vi "三角函數功能.vi"() -> ()   [LabVIEW 2015]
panel:
  out "angle":dbl(graph)
  out "Numeric":i32
  out "Boolean":bool
  out "radian":dbl(graph)
  in  "angle Control 2":dbl
  in  "三角函數":u16(ring)=1 items=["sin", "cos", "tan", "csc", "sec", "cot"]
  out "res angle(num)":dbl
  in  "Stop Button":bool
  out "換算角度 angle (num)":dbl
  in  "angle Control":dbl(slide) scale=0.0..360.0
  out "res radian(num)":dbl
  out "res angle(gauge)":dbl(knob)
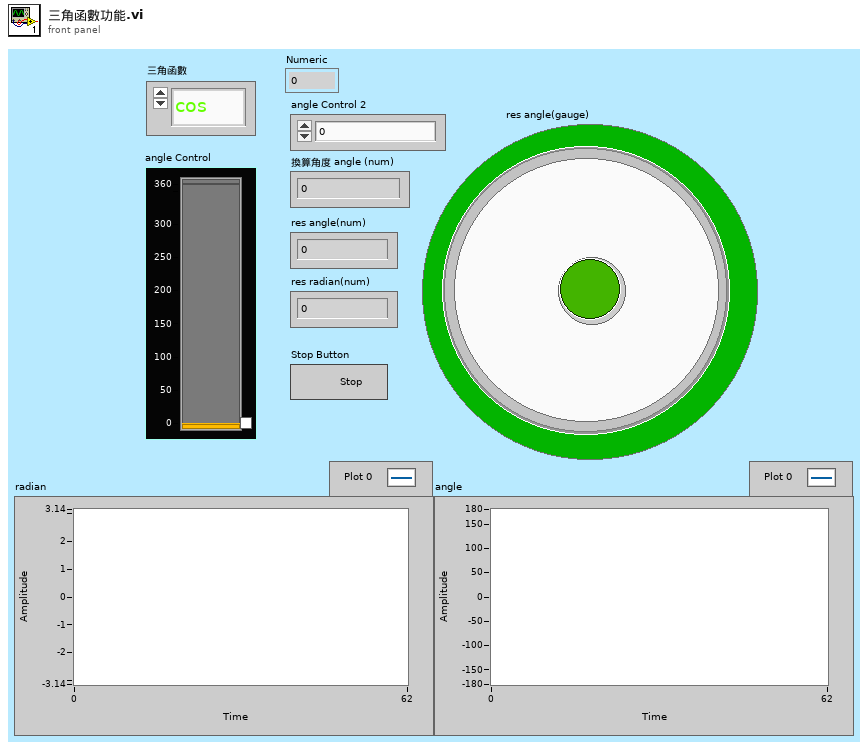
[diagram p1: front panel]
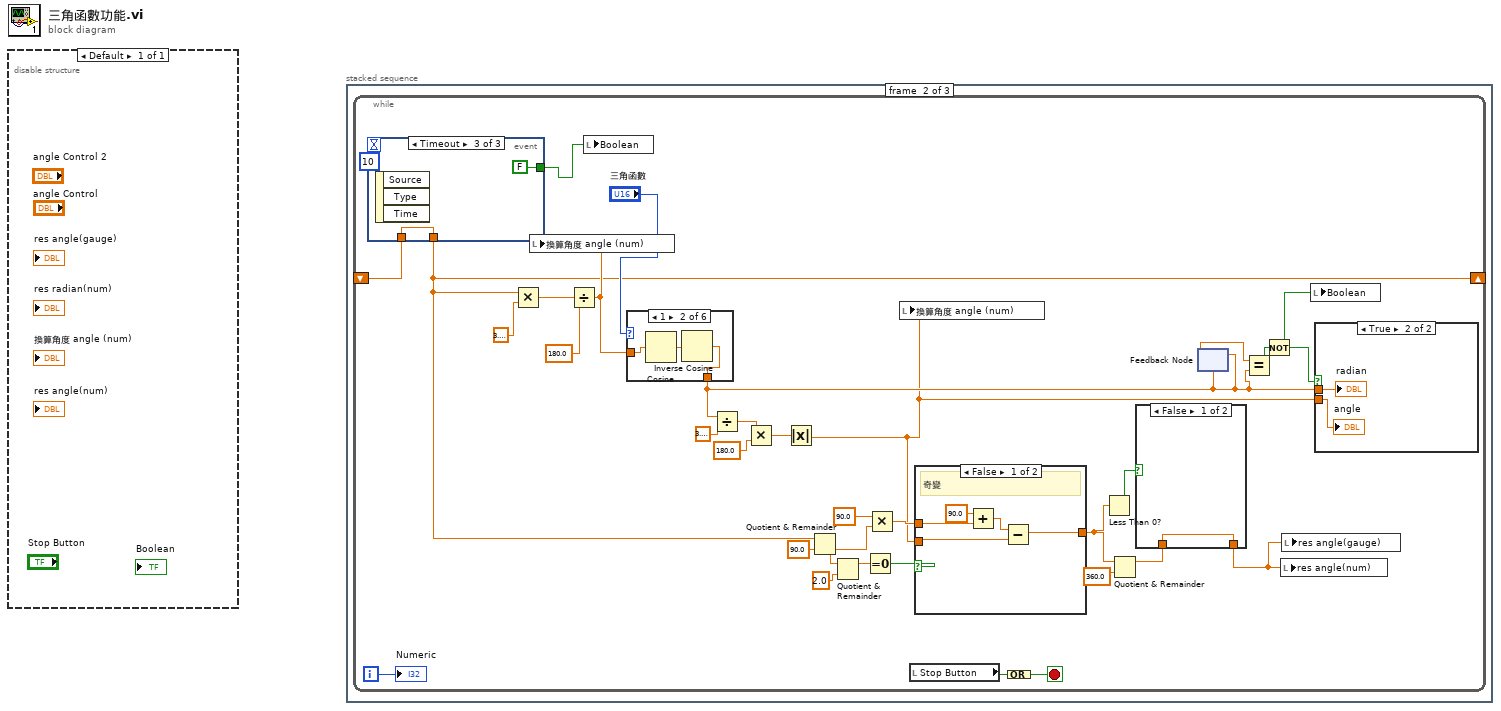
[diagram p0: block diagram]
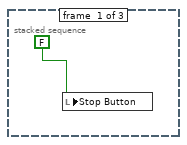
[diagram p2: hidden frame]
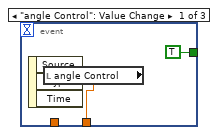
[diagram p3: hidden frame]
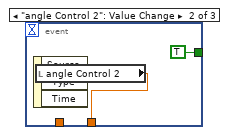
[diagram p4: hidden frame]
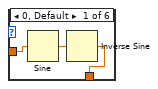
[diagram p6: hidden frame]
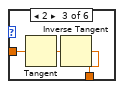
[diagram p7: hidden frame]
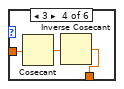
[diagram p8: hidden frame]
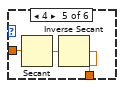
[diagram p9: hidden frame]
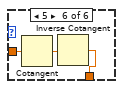
[diagram p10: hidden frame]
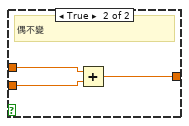
[diagram p12: hidden frame]
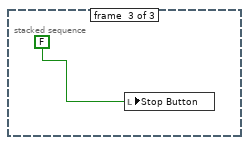
[diagram p13: hidden frame]
diagram:
  n1 = disable-structure shown="Default" {
    frame Enabled {
    }
  }
  n2 = stacked-sequence {
    frame #0 {
      n3 = local write "Stop Button"(FALSE ("Stop Button")) -> ()
    }
    frame #1 {
      n4 = while {
        shift-right: [w4] -> _
        shift-left: _ -> [w3]
        i -> [w6]
        stop <- w34 stop-if-true
        n5 = event shown="[2] Timeout" {
          selector: _ -> [_ _ _]
          dyn-events: _ -> [_ _ _]
          timeout: 10 -> [_ _ _]
          tunnel: [w36 w38 w39] -> w4
          tunnel: [TRUE TRUE FALSE] -> w5
          tunnel: w3 -> [_ _ w39]
          event "angle Control": Value Change {
            n6 = event-data() -> ()  [unwired: 1 in, 3 out]
            n7 = local read "angle Control"() -> (w36:dbl)
          }
          event "angle Control 2": Value Change {
            n8 = event-data() -> ()  [unwired: 1 in, 3 out]
            n9 = local read "angle Control 2"() -> (w38:dbl)
          }
          event Timeout {
            n10 = event-data() -> ()  [unwired: 1 in, 3 out]
          }
        }
        n11 = Multiply(x=w4, y=3.141592653589793) -> (x*y=w29:dbl)
        n12 = Divide(x=w29, y=180.0) -> (x/y=w27:dbl)
        n13 = local write "換算角度 angle (num)"(w27) -> ()
        n14 = local write "Boolean"(w5) -> ()
        n15 = case shown="1" "三角函數" {
          tunnel: w27 -> [w45 w47 w51 w54 w57 w60]
          tunnel: [w44 w46 w49 w52 w55 w58] -> w10
          frame 0, Default {
            n16 = Sine(x=w45) -> (sin(x)=w43:dbl)
            n17 = Inverse Sine(1:w43) -> (0:w44:dbl)
          }
          frame 1 {
            n18 = Cosine(x=w47) -> (cos(x)=w48:dbl)
            n19 = Inverse Cosine(1:w48) -> (0:w46:dbl)
          }
          frame 2 {
            n20 = Tangent(1:w51) -> (0:w50:dbl)
            n21 = Inverse Tangent(1:w50) -> (0:w49:dbl)
          }
          frame 3 {
            n22 = Cosecant(1:w54) -> (0:w53:dbl)
            n23 = Inverse Cosecant(1:w53) -> (0:w52:dbl)
          }
          frame 4 {
            n24 = Secant(1:w57) -> (0:w56:dbl)
            n25 = Inverse Secant(1:w56) -> (0:w55:dbl)
          }
          frame 5 {
            n26 = Cotangent(1:w60) -> (0:w59:dbl)
            n27 = Inverse Cotangent(1:w59) -> (0:w58:dbl)
          }
        }
        n28 = Divide(x=w10, y=3.141592653589793) -> (x/y=w31:dbl)
        n29 = Multiply(x=w31, y=180.0) -> (x*y=w18:dbl)
        n30 = Absolute Value(x=w18) -> (abs(x)=w2:dbl)
        n31 = Quotient & Remainder(x=w4, y=90.0) -> (floor(x/y)=w21:dbl)  [unwired: 1 out]
        n32 = Quotient & Remainder(x=w21, y=2.0) -> (x-y*floor(x/y)=w24:dbl)  [unwired: 1 out]
        n33 = Equal To 0?(x=w24) -> (x = 0?=w20:bool)
        n34 = Multiply(x=90.0, y=w21) -> (x*y=w19:dbl)
        n35 = local write "換算角度 angle (num)"(w2) -> ()
        n36 = local read "Stop Button"() -> (w33:bool)
        n37 = case shown="False" w20 {
          tunnel: w19 -> [w66 w70]
          tunnel: w2 -> [w63 w69]
          tunnel: [w67 w68] -> w16
          frame False {
            # "奇變"
            n38 = Add(x=90.0, y=w66) -> (x+y=w64:dbl)
            n39 = Subtract(x=w64, y=w63) -> (x-y=w67:dbl)
          }
          frame True {
            # "偶不變"
            n40 = Add(x=w70, y=w69) -> (x+y=w68:dbl)
          }
        }
        n41 = Compound Arithmetic op=OR(w33) -> (w34:bool)
        n42 = Less Than 0?(x=w16) -> (x < 0?=w14:bool)
        n43 = Quotient & Remainder(x=w16, y=360.0) -> (x-y*floor(x/y)=w15:dbl)  [unwired: 1 out]
        n44 = case shown="False" w14 {
          tunnel: [w61 w62] -> w12
          tunnel: w15 -> [w61 w62]
          frame False {
          }
          frame True {
          }
        }
        n45 = feedback-in #1(w10) -> ()
        n46 = feedback #1(w10) -> (w11:dbl)
        n47 = Equal?(x=w11, y=w10) -> (x = y?=w9:bool)
        n48 = Not(x=w9) -> (.not. x?=w8:bool)
        n49 = local write "res angle(num)"(w12) -> ()
        n50 = local write "res angle(gauge)"(w12) -> ()
        n51 = local write "Boolean"(w8) -> ()
        n52 = case shown="True" w8 {
          tunnel: w10 -> [_ w42]
          tunnel: w2 -> [_ w41]
          frame False {
          }
          frame True {
            "radian" <- w42
            "angle" <- w41
          }
        }
        "Numeric" <- w6
      }
    }
    frame #2 {
      n53 = local write "Stop Button"(FALSE ("Stop Button")) -> ()
    }
  }
